vi "QPSK Demodulation.vi"() -> (0 "size(s)":i32, 1 "Output bits":dbl[](array[numeric]), 2 "Constellation graph":cluster{"Y":dbl[], "Y":dbl[]}[](graph), 3 "Even bits":dbl[](graph), 4 "output bits graph":dbl[](graph), 5 "Odd bits":dbl[](graph))   [LabVIEW 2026]
panel:
  in  "Array 2":dynamicdata[](array[waveform])
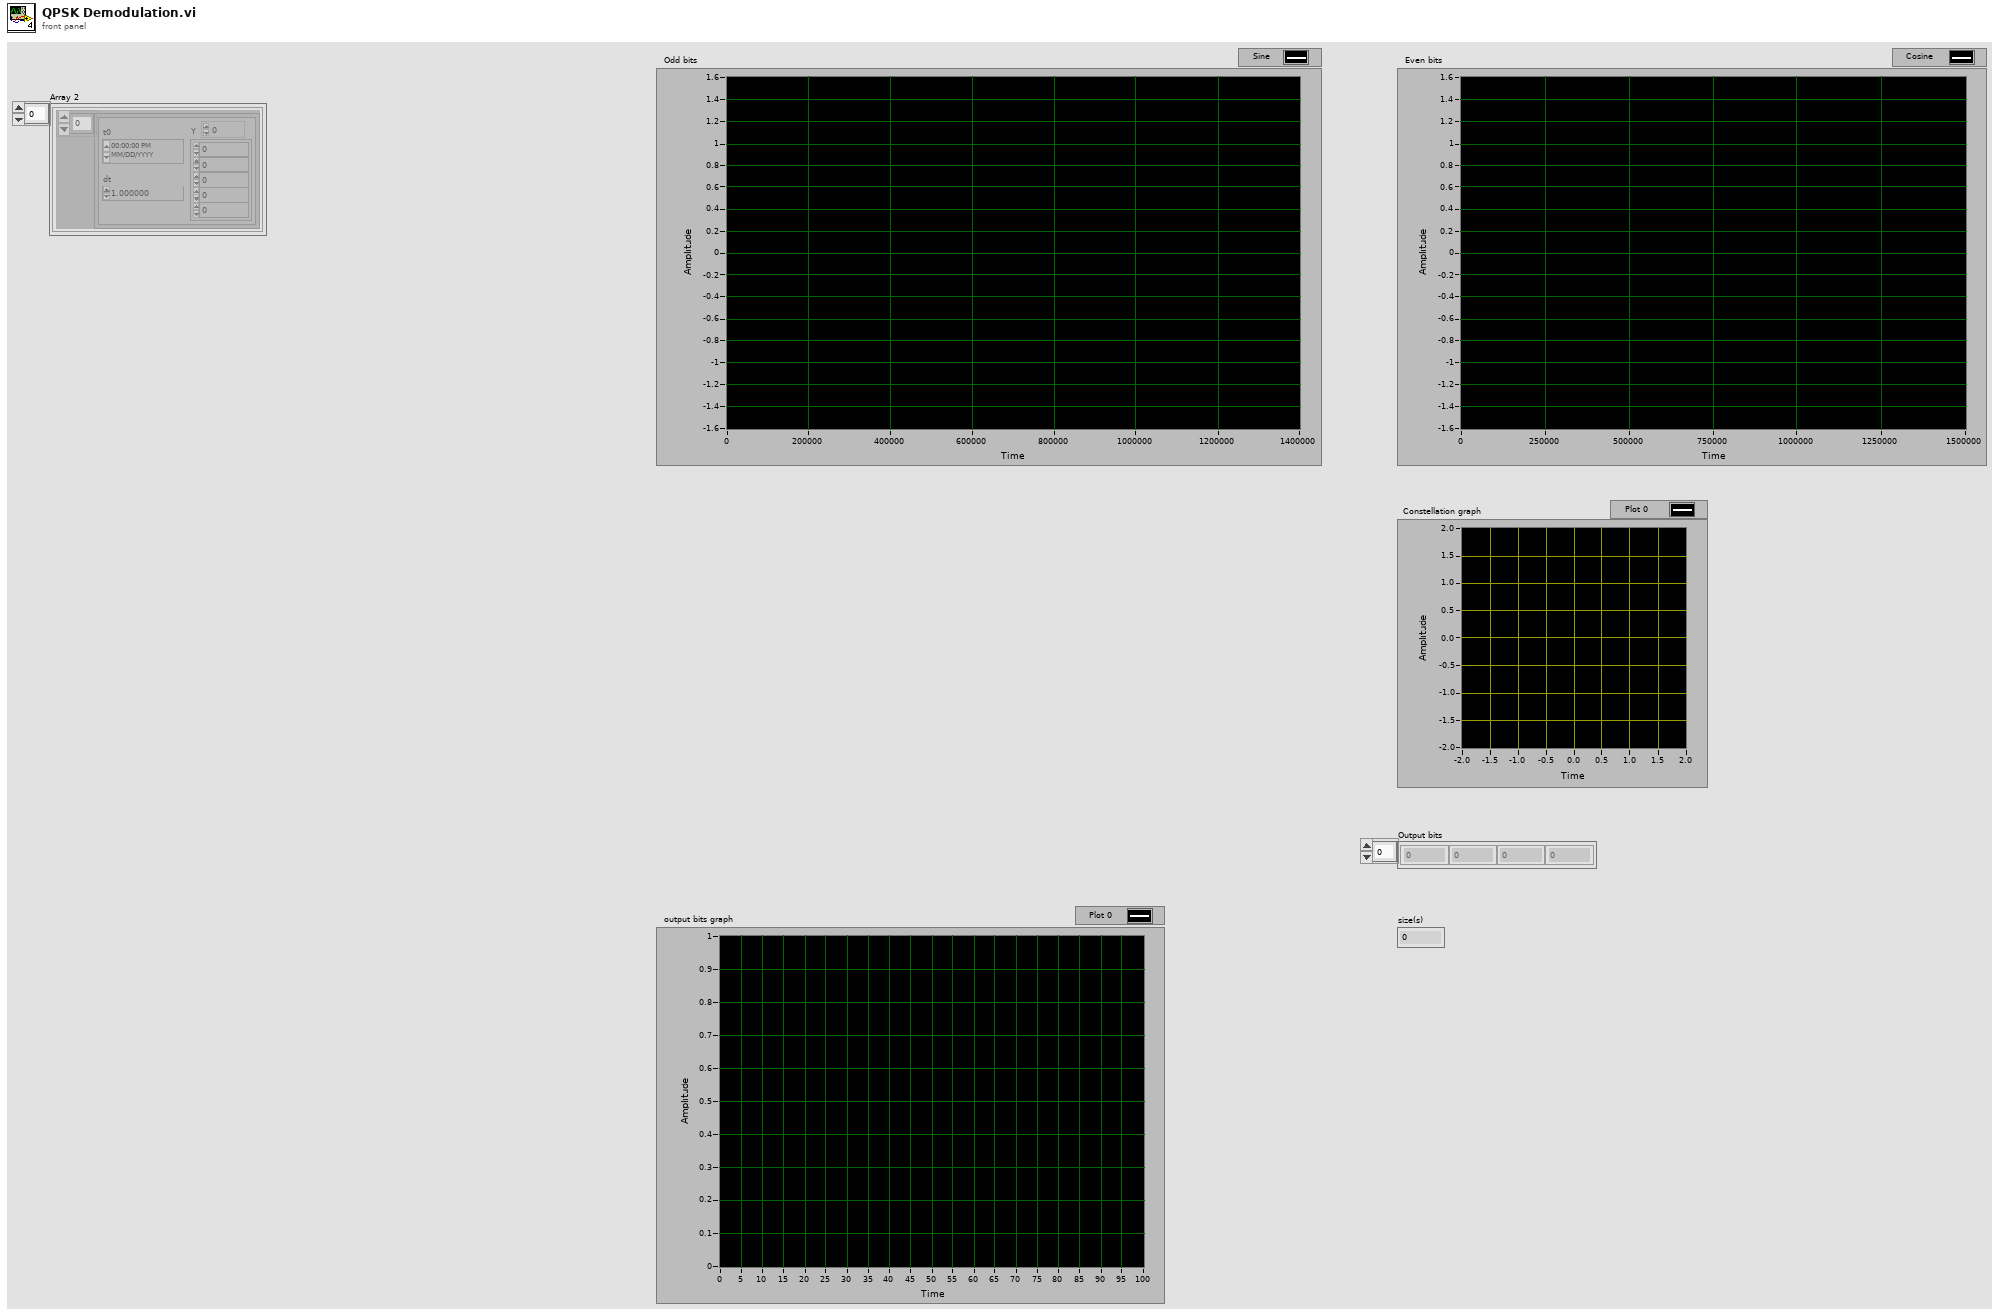
[diagram p1: front panel]
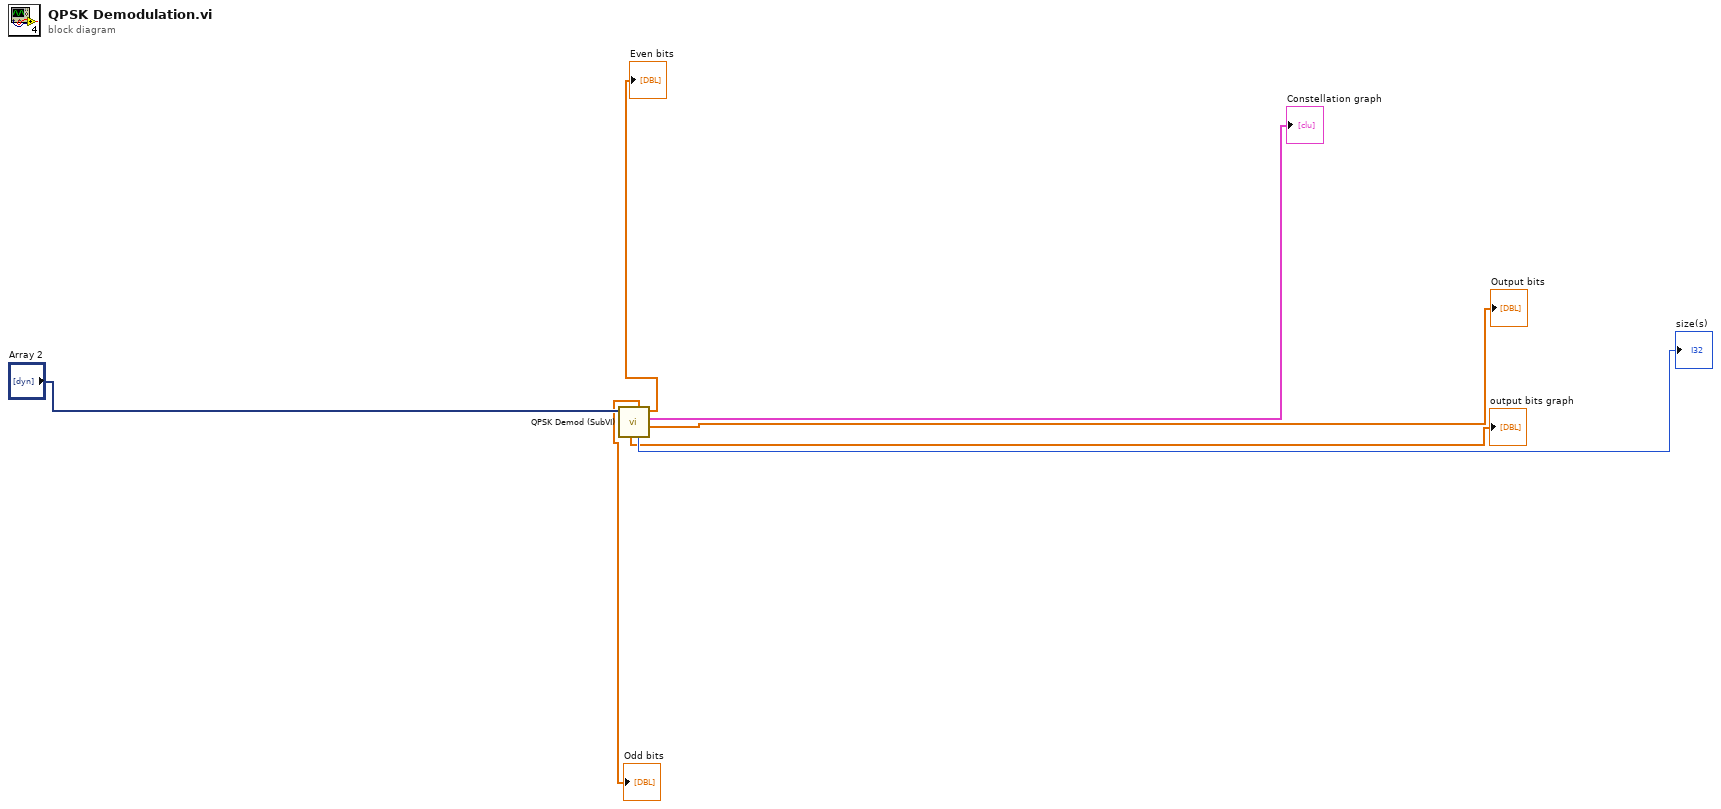
[diagram p0: block diagram]
diagram:
  n1 = call "QPSK Demod (SubVI).vi"("Array in"="Array 2") -> ("Output bits"=→"Output bits":dbl[], "Constellation graph"=→"Constellation graph":cluster{"Y":dbl[], "Y":dbl[]}[], "Even bits"=→"Even bits":dbl[], "size(s)"=→"size(s)":i32, "Odd bits"=→"Odd bits":dbl[], "output bits graph"=→"output bits graph":dbl[])  [unwired: 5 in]
